vi "Helmholtz2D_FEM_Assemble_Mass Mtrx.vi"(9 "area":dbl, 10 "Tri Y":dbl[](array[numeric]), 11 "Tri X":dbl[](array[numeric])) -> (3 "Mass Mtrx":dbl[][](array[numeric]))   [LabVIEW 2017, in "NI_PDE.lvlib"]
uses:
  <vilib>/gmath/NI_PDE.lvlib
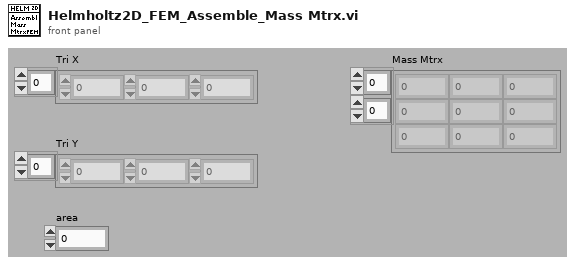
[diagram p1: front panel]
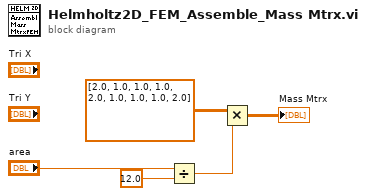
[diagram p0: block diagram]
diagram:
  n1 = Divide(x="area", y=12.0) -> (x/y=w1:dbl)
  n2 = Multiply(x=dbl[][] [[2.0, 1.0, 1.0], [1.0, 2.0, 1.0], [1.0, 1.0, 2.0]] ("Mass Mtrx"), y=w1) -> (x*y=→"Mass Mtrx":dbl[][])
